vi "Control Discrete Relay.vi"(0 "Control":T1, 2 "State":bool, 5 "error in":errorcluster, 6 "Device Name":string="Dev1") -> (19 "error out":errorcluster={"status"=TRUE, "code"=-200220, "source"="DAQmx Create Channel (DO-Digital Output).vi:2<append>\n<B>Device Specified: </B>Dev1\n\n<B>Task Name: </B>_unnamedTask<0>"})   [LabVIEW 2015]
uses:
  Discrete Controls.ctl
panel:
  out "State":bool
  # "K1 Not Used\nK2 Not Used\nK3 Not Used\n---->K4 Interlock  :: P1.3\n\nK5 Not Used\nK6 Not Used\n\nK7 Not Used\nK8 Not Used\nK9 REF-2.5        :: P2.0\nK10 +3.3V         :: P2.1\nK11 +5.2V         :: P2.2\nK12 +5.2VA       :: P2.3\nK13 -5.2VA        :: P2.4\nK14 +1.6V          :: P2.5\n\nK15    SPARE\n---->K16   VBAT :: P2.7"
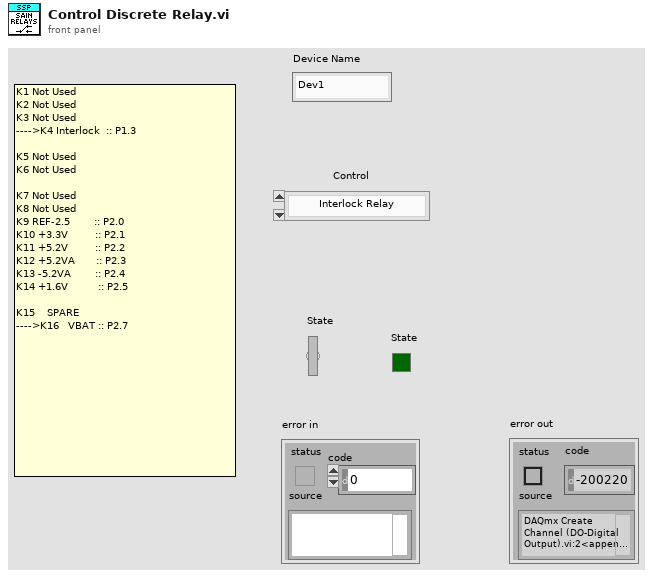
[diagram p1: front panel]
types:
  T1 = typedef "Discrete Controls.ctl" = enum16{"Interlock Relay", "VBAT UUT Power", "Pneumatic"}
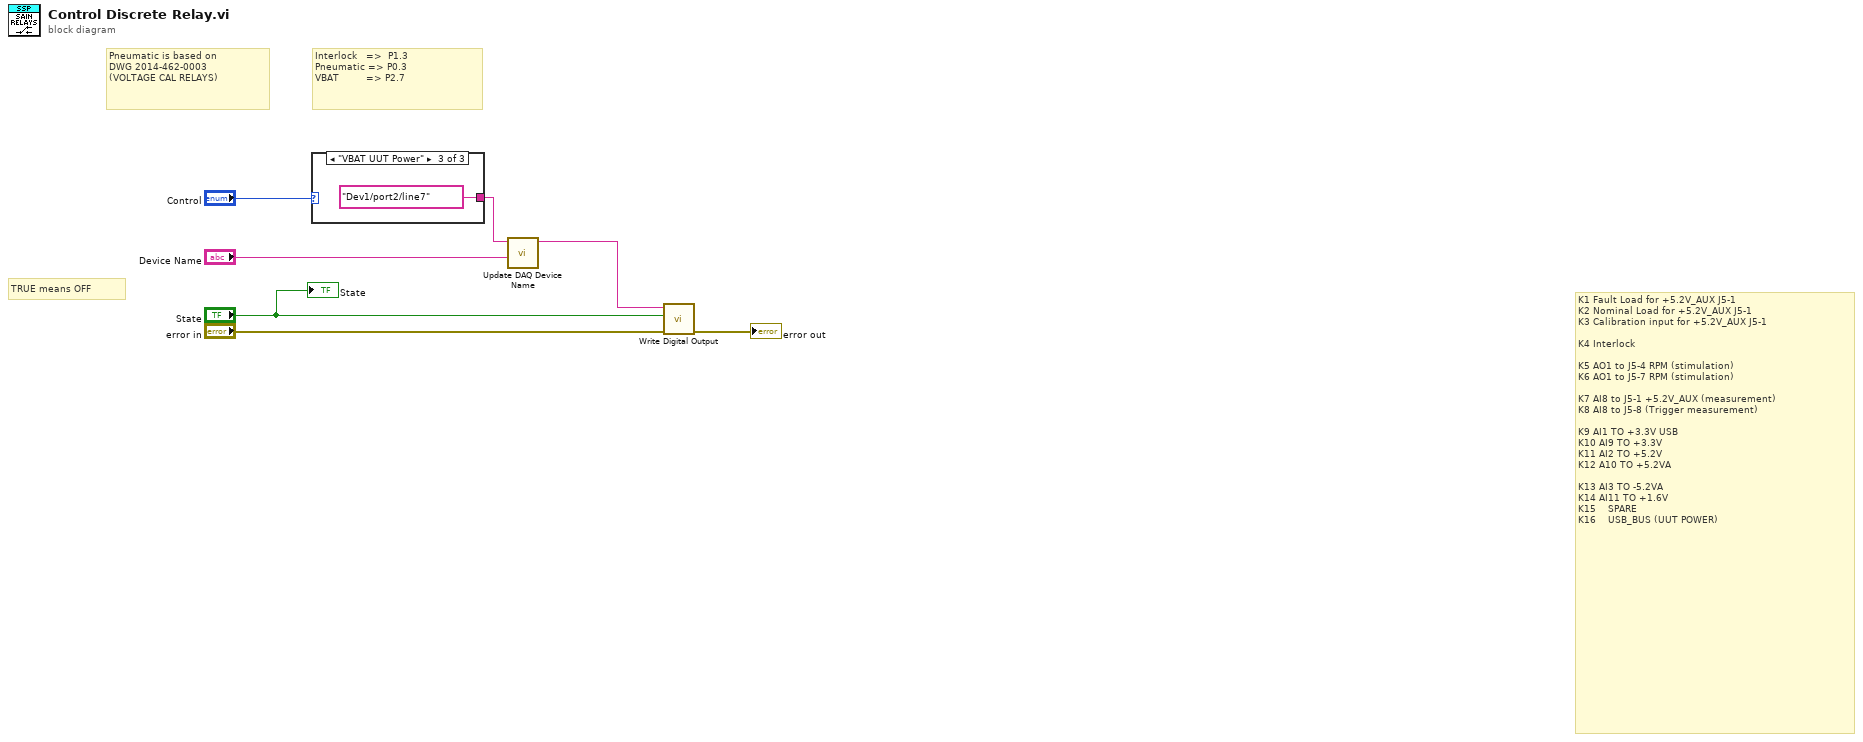
[diagram p0: block diagram]
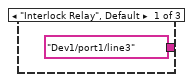
[diagram p2: hidden frame]
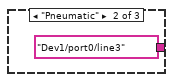
[diagram p3: hidden frame]
diagram:
  # "TRUE means OFF"
  # "Pneumatic is based on \nDWG 2014-462-0003\n(VOLTAGE CAL RELAYS)"
  # "Interlock   =>  P1.3 \nPneumatic => P0.3 \nVBAT         => P2.7"
  # "K1 Fault Load for +5.2V_AUX J5-1 \nK2 Nominal Load for +5.2V_AUX J5-1 \nK3 Calibration input for +5.2V_AUX J5-1 \n\nK4 Interlock\n\nK5 AO1 to J5-4 RPM (stimulation)\nK6 AO1 to J5-7 RPM (stimulation)\n\nK7 AI8 to J5-1 +5.2V_AUX (measurement)\nK8 AI8 to J5-8 (Trigger measurement)\n\nK9 AI1 TO +3.3V USB\nK10 AI9 TO +3.3V\nK11 AI2 TO +5.2V\nK12 A10 TO +5.2VA\n\nK13 AI3 TO -5.2VA\nK14 AI11 TO +1.6V\nK15    SPARE\nK16    USB_BUS (UUT POWER)"
  n1 = case shown="\"VBAT UUT Power\"" "Control" {
    tunnel: ["Dev1/port1/line3" "Dev1/port0/line3" "Dev1/port2/line7"] -> w4
    frame "Interlock Relay", Default {
    }
    frame "Pneumatic" {
    }
    frame "VBAT UUT Power" {
    }
  }
  n2 = call "Update DAQ Device Name.vi"("Device Name"="Device Name", "Lines in (String)"=w4) -> ("Lines out (DAQmx Physical Channels)"=w3:tag)  [unwired: 9 in]
  n3 = call "Write Digital Output.vi"("error in"="error in", "data"="State", "Write lines"=w3) -> ("error out"=→"error out":errorcluster)  [unwired: 8 in]
  "State" <- "State"
